vi "add_to_status_list.vi"(2 "string":string, 3 "ListBox in":refnum<vi>) -> ()   [LabVIEW 2015]
doc: "adds the string to the status listbox\nand scrolsl the listbox"
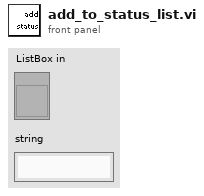
[diagram p1: front panel]
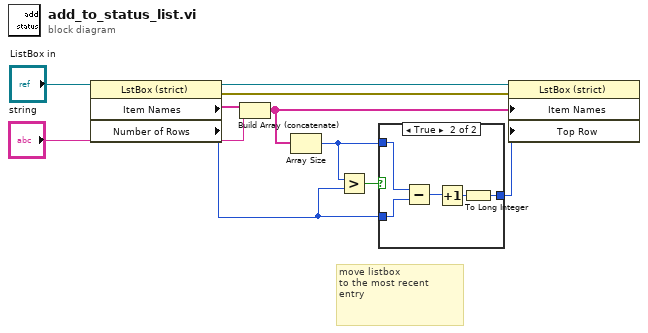
[diagram p0: block diagram]
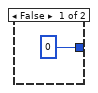
[diagram p2: hidden frame]
diagram:
  # "move listbox\nto the most recent\nentry"
  n1 = property on="Property Node" class="LstBox (strict)"(reference="ListBox in") -> (reference out=w6:refnum<vi>, error out=w10:errorcluster, "Item Names"=w8:string[], "Number of Rows"=w2:u32)  [unwired: 1 in]
  n2 = Build Array (concatenate)(w8, "string") -> (w5:string[])
  n3 = Array Size(array=w5) -> (size(s)=w3:i32)
  n4 = Greater?(x=w3, y=w2) -> (0:w4:bool)
  n5 = case shown="True" w4 {
    tunnel: [0 w13] -> w1
    tunnel: w3 -> [_ w15]
    tunnel: w2 -> [_ w14]
    frame False {
    }
    frame True {
      n6 = Subtract(x=w15, y=w14) -> (x-y=w16:u32)
      n7 = Increment(x=w16) -> (x+1=w12:u32)
      n8 = To Long Integer(number=w12) -> (32bit integer=w13:i32)
    }
  }
  n9 = property on="Property Node" class="LstBox (strict)"(reference=w6, error in=w10, "Item Names"=w5, "Top Row"=w1) -> ()  [unwired: 2 out]
